vi "Read System ADC.vi"(8 "error in (no error)":errorcluster, 11 "DCM-DSI-HW in":refnum<class "DCM-DSI.lvclass">) -> (0 "error out":errorcluster, 2 "System ADC":T1 {"Fan [V]" format="%#_3p"; "Primary B1B2 [V]" format="%#_3p"; "Primary B3B4 [V]" format="%#_3p"; "Primary A3A4 [V]" format="%#_3p"; "Primary A1A2 [V]" format="%#_3p"; "MPRD [V]" format="%#_3p"; "Ext HV B [V]" format="%#_3p"; "Ext HV A [V]" format="%#_3p"; "Pump Zener B [V]" format="%#_3p"; "Pump Zener A [V]" format="%#_3p"; "DI Zener B [V]" format="%#_3p"; "DI Zener A [V]" format="%#_3p"; "Key [V]" format="%#_3p"; "DRVP [V]" format="%#_3p"; "Battery [V]" format="%#_3p"; "FET Driver [V]" format="%#_3p"; "Secondary B1B2 [V]" format="%#_3p"; "Secondary B3B4 [V]" format="%#_3p"; "Secondary A3A4 [V]" format="%#_3p"; "Secondary A1A2 [V]" format="%#_3p"; "Primary Range [V]" format="%#_3p"; "Temp Boost B [C]" format="%#_3p"; "Temp Primary A [C]" format="%#_3p"; "Temp Secondary A [C]" format="%#_3p"; "Temp Fan Intake [C]" format="%#_3p"; "Temp CPU [C]" format="%#_3p"; "Temp DI Zener B [C]" format="%#_3p"; "Temp DI B [C]" format="%#_3p"; "Temp DI Zener A [C]" format="%#_3p"; "Temp DI A [C]" format="%#_3p"; "Temp HH 7-12 [C]" format="%#_3p"; "Temp HH 1-6 [C]" format="%#_3p"; "AI 12 [V]" format="%#_3p"; "AI 11 [V]" format="%#_3p"; "AI 10 [V]" format="%#_3p"; "AI 9 [V]" format="%#_3p"; "AI 8 [V]" format="%#_3p"; "AI 7 [V]" format="%#_3p"; "AI 6 [V]" format="%#_3p"; "AI 5 [V]" format="%#_3p"; "AI 4 [V]" format="%#_3p"; "AI 3 [V]" format="%#_3p"; "AI 2 [V]" format="%#_3p"; "AI 1 [V]" format="%#_3p"}, 3 "DCM-DSI-HW out":refnum<class "DCM-DSI.lvclass">)   [LabVIEW 2016, in "DCM-DSI.lvclass"]
uses:
  DCM-DSI.lvclass
  <vilib>/Powertrain Controls/Device Drivers/DCM/Rev0/RT/System ADC.ctl
  DCM-DSI.lvclass/DCM-DSI.ctl
  <vilib>/Powertrain Controls/Device Drivers/DCM/Rev0/RT/DCM - RT.lvclass
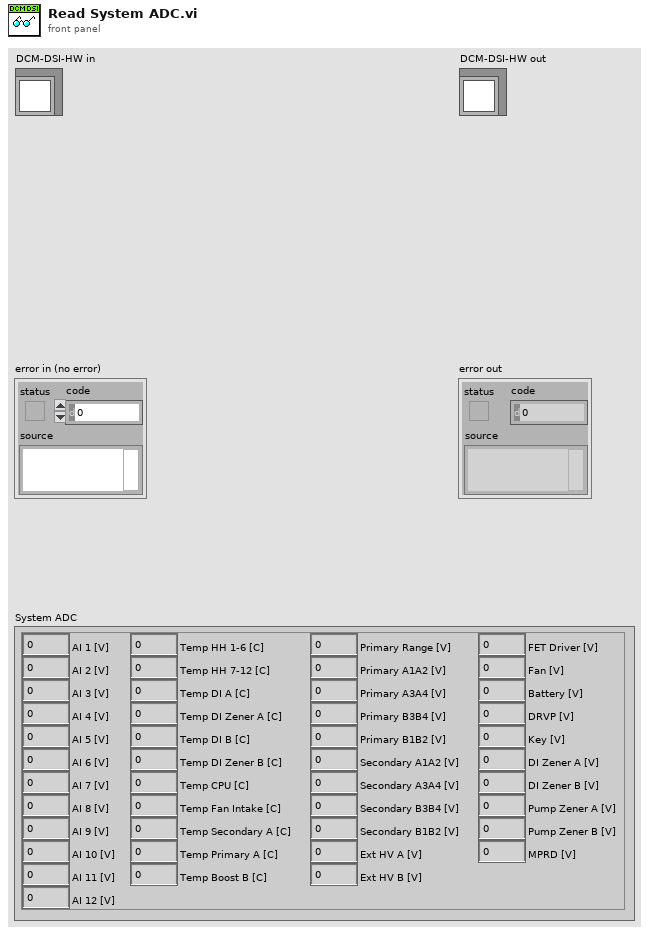
[diagram p1: front panel]
types:
  T1 = typedef "DCM - RT.lvclass/System ADC.ctl" = cluster{"AI 1 [V]":sgl, "AI 2 [V]":sgl, "AI 3 [V]":sgl, "AI 4 [V]":sgl, "AI 5 [V]":sgl, "AI 6 [V]":sgl, "AI 7 [V]":sgl, "AI 8 [V]":sgl, "AI 9 [V]":sgl, "AI 10 [V]":sgl, "AI 11 [V]":sgl, "AI 12 [V]":sgl, "Temp HH 1-6 [C]":sgl, "Temp HH 7-12 [C]":sgl, "Temp DI A [C]":sgl, "Temp DI Zener A [C]":sgl, "Temp DI B [C]":sgl, "Temp DI Zener B [C]":sgl, "Temp CPU [C]":sgl, "Temp Fan Intake [C]":sgl, "Temp Secondary A [C]":sgl, "Temp Primary A [C]":sgl, "Temp Boost B [C]":sgl, "Primary Range [V]":sgl, "Primary A1A2 [V]":sgl, "Primary A3A4 [V]":sgl, "Primary B3B4 [V]":sgl, "Primary B1B2 [V]":sgl, "Secondary A1A2 [V]":sgl, "Secondary A3A4 [V]":sgl, "Secondary B3B4 [V]":sgl, "Secondary B1B2 [V]":sgl, "Ext HV A [V]":sgl, "Ext HV B [V]":sgl, "FET Driver [V]":sgl, "Fan [V]":sgl, "Battery [V]":sgl, "DRVP [V]":sgl, "Key [V]":sgl, "DI Zener A [V]":sgl, "DI Zener B [V]":sgl, "Pump Zener A [V]":sgl, "Pump Zener B [V]":sgl, "MPRD [V]":sgl}
  T2 = typedef "DCM - RT.lvclass/System State.ctl" = cluster{"System ADC":T1, "IO Lock":bool, "HH Mode Config Error":bool, "Fan Speed 1 [RPM]":sgl, "Fan Speed 2 [RPM]":sgl, "Firmware Major Rev":u16, "Firmware Minor Rev":u16, "Internal Fault":T3, "Fault Value":dbl}
  T3 = typedef "DCM - RT.lvclass/Internal Fault.ctl" = enum32{"None", "Temp HH 1-6", "Temp HH 7-12", "Temp DI A", "Temp DI Zener A", "Temp DI B", "Temp DI Zener B", "Temp Intake", "Temp Primary A", "Temp Secondary A", "Temp Boost B", "Temp CPU", "Low Battery", "Inrush Protection", "A Run Enable", "B Run Enable", "Fan Speed"}
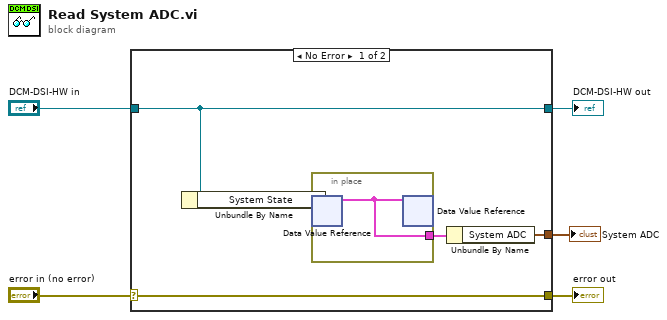
[diagram p0: block diagram]
diagram:
  n1 = case shown="No Error" "error in (no error)" {
    selector: "error in (no error)" -> [w10 w13]
    tunnel: [w10 w13] -> w4
    tunnel: [w8 w12] -> w2
    tunnel: "DCM-DSI-HW in" -> [w8 w12]
    tunnel: [w6 _] -> w1
    frame No Error {
      n2 = Unbundle By Name(w8) -> ("System State"=w9:refnum<data-value>)
      n3 = in-place {
        in-place-border: [w11] -> w7
        n4 = in-place-dvr #1(w9) -> (w11:T2)  [unwired: 1 out]
        n5 = in-place-dvr #1(w11) -> ()  [unwired: 2 out]
      }
      n6 = Unbundle By Name(w7) -> ("System ADC"=w6:T1)
    }
    frame Error {
    }
  }
  "error out" <- w4
  "DCM-DSI-HW out" <- w2
  "System ADC" <- w1
